vi "Read Build Data.vi"(0 "Build Named Build Specification Data in":refnum<class "Build Named Build Specification Data.lvclass">, 11 "error in (no error)":errorcluster) -> (4 "Build Named Build Specification Data out":refnum<class "Build Named Build Specification Data.lvclass">, 6 "Generated files":path[](array[path]), 8 "Build Specification Name":string, 10 "Target Name":string, 15 "error out":errorcluster)   [LabVIEW 2019, in "ProjectBuilder.lvlib" / "Build Named Build Specification Data.lvclass"]
doc: "Read private data."
uses:
  Build Named Build Specification Data.lvclass
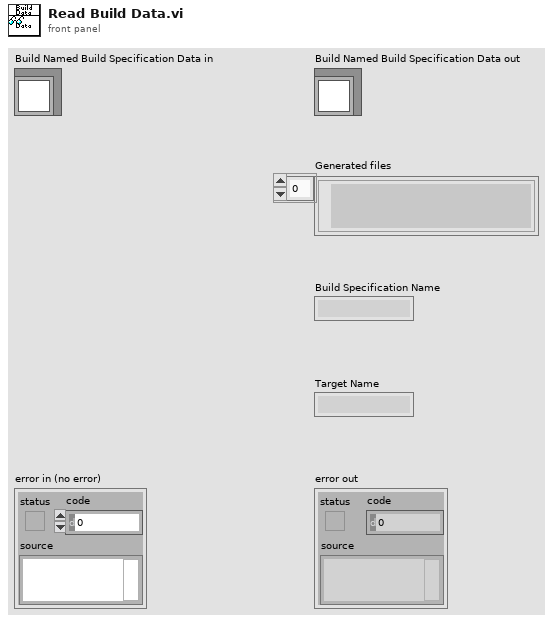
[diagram p1: front panel]
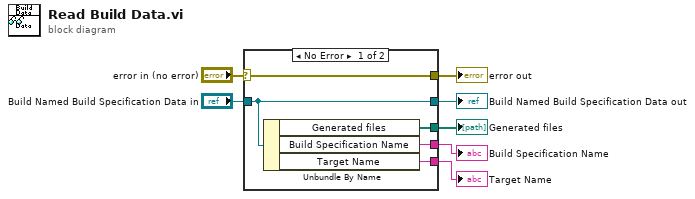
[diagram p0: block diagram]
diagram:
  n1 = case shown="No Error" "error in (no error)" {
    selector: "error in (no error)" -> [w12 w13]
    tunnel: [w12 w13] -> w6
    tunnel: [w11 w14] -> w4
    tunnel: "Build Named Build Specification Data in" -> [w11 w14]
    tunnel: [w10 _] -> w3
    tunnel: [w9 _] -> w2
    tunnel: [w8 _] -> w1
    frame No Error {
      n2 = Unbundle By Name(w11) -> ("Generated files"=w10:path[], "Build Specification Name"=w9:string, "Target Name"=w8:string)
    }
    frame Error {
    }
  }
  "error out" <- w6
  "Build Named Build Specification Data out" <- w4
  "Generated files" <- w3
  "Build Specification Name" <- w2
  "Target Name" <- w1
